vi "myRIO_BRig_RT_dataLC_Selection_Count_NS_l1.vi"() -> (2 "output_Selection_Count_NS_l1":i32)   [LabVIEW 2014]
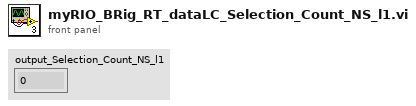
[diagram p1: front panel]
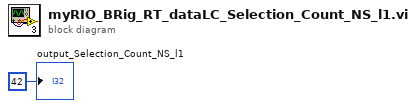
[diagram p0: block diagram]
diagram:
  "output_Selection_Count_NS_l1" <- 42 ("output_iBlock")
